vi "Delacor_lib_QMH_Check Loop Error.vi"(6 "Error Message Name (\"Error\")":string="Error", 9 "Ignore Errors":i32[](array[numeric]), 10 "error to process":errorcluster, 11 "Message Queue in":refnum<class "Delacor_lib_QMH_Message Queue.lvclass">) -> (2 "Enqueued Error?":bool, 3 "Message Queue out":refnum<class "Delacor_lib_QMH_Message Queue.lvclass">)   [LabVIEW 2024, in "Delacor_lib_QMH_Message Queue.lvclass"]
doc: "Check the 'error to process' to see if its code value matches any of the values in the 'Ignore Errors' array. If so, do nothing. If not, send an \"Error\" message containing the error data to the Message Handling Loop for further processing.\n____\nDQMH Framework: Palette 7.1.0.1503\nCopyright (c) 2025, DQMH Consortium"
uses:
  Delacor_lib_QMH_Message Queue.lvclass
  Delacor_lib_QMH_Message Queue.lvclass/Delacor_lib_QMH_Message Queue.ctl
  <vilib>/Delacor/Delacor QMH/Libraries/Message Queue_class/Delacor_lib_QMH_Enqueue Message (Single).vi
  Delacor_lib_QMH_Get Error Debug.vi
  Delacor_lib_QMH_Set Error Debug.vi
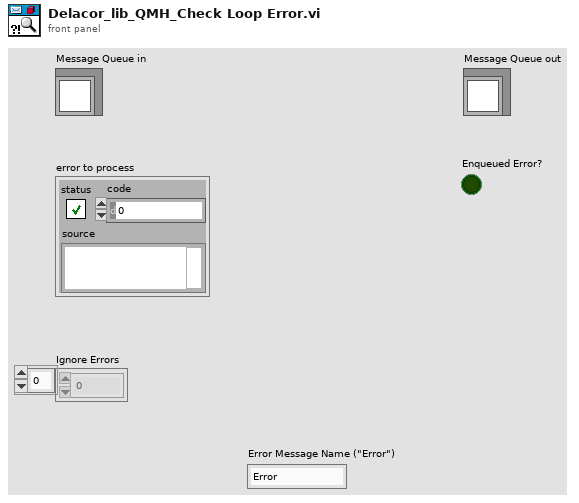
[diagram p1: front panel]
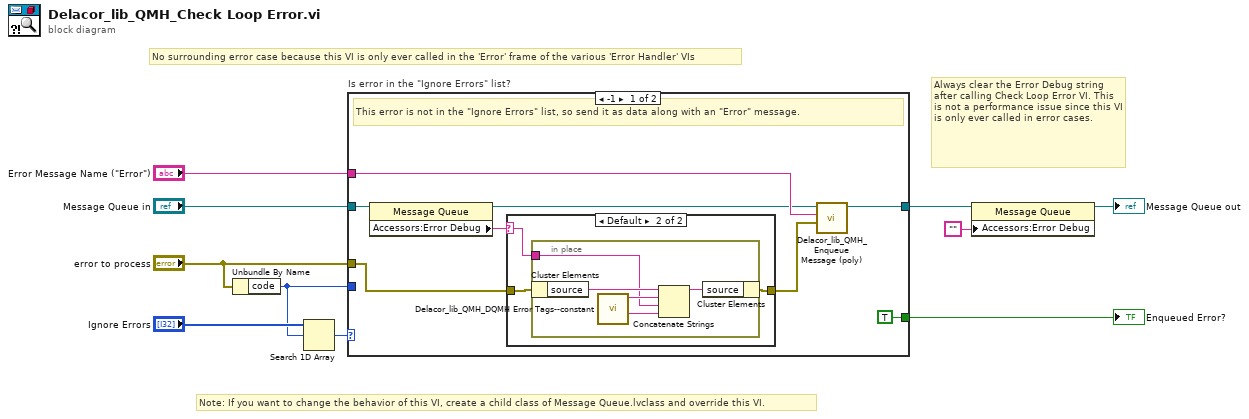
[diagram p0: block diagram]
diagram:
  # "No surrounding error case because this VI is only ever called in the 'Error' frame of the various 'Error Handler' VIs"
  # "Always clear the Error Debug string after calling Check Loop Error VI. This is not a performance issue since this VI is only ever called in error cases."
  # "Note: If you want to change the behavior of this VI, create a child class of Message Queue.lvclass and override this VI."
  n1 = Unbundle By Name("error to process") -> ("code"=w1:i32)
  n2 = Search 1D Array(1D array="Ignore Errors", element=w1) -> (index of element=w2:i32)  [unwired: 1 in]
  n3 = case "Is error in the \"Ignore Errors\" list?" shown="-1" w2 {
    tunnel: "error to process" -> [w14 _]
    tunnel: "Message Queue in" -> [w18 w28]
    tunnel: w1 -> [_ _]
    tunnel: [TRUE _] -> w7
    tunnel: [w16 w28] -> w6
    tunnel: "Error Message Name (\"Error\")" -> [w15 _]
    frame -1 {
      # "This error is not in the \"Ignore Errors\" list, so send it as data along with an \"Error\" message."
      n4 = property class="Message Queue"(reference=w18) -> (reference out=w11:refnum<class "Delacor_lib_QMH_Message Queue.lvclass">, "Accessors:Error Debug"=w12:string)  [unwired: 1 in, 1 out]
      n5 = case shown="Default" w12 {
        selector: w12 -> [_ w20]
        tunnel: w14 -> [w19 w22]
        tunnel: [w19 w21] -> w13
        frame "" {
          # "Don't add Error Debug string to error source string if it is empty."
        }
        frame Default {
          n6 = in-place {
            in-place-border: w20 -> [w24]
            n7 = in-place-cluster #1(w22) -> ("source"=w27:string)
            n8 = call <vilib>:"Delacor_lib_QMH_DQMH Error Tags--constant.vi"() -> ("Close Tag"=w23:string, "Open Tag"=w25:string)  [unwired: 10 in]
            n9 = Concatenate Strings(w27, w25, w24, w23) -> (w26:string)
            n10 = in-place-cluster #1("source"=w26) -> (w21:errorcluster)
          }
        }
      }
      n11 = call-poly <vilib>:"Delacor_lib_QMH_Enqueue Message (poly).vi"("Message Data"=w13, "Message"=w15, "Message Queue in"=w11) -> ("Message Queue out"=w16:refnum<class "Delacor_lib_QMH_Message Queue.lvclass">)  [unwired: 7 in, 1 out]
    }
    frame Default {
      # "This error is is in the \"Ignore Errors\" list, so do not send it for processing."
    }
  }
  "Enqueued Error?" <- w7
  n12 = property class="Message Queue"(reference=w6, "Accessors:Error Debug"="") -> (reference out=→"Message Queue out":refnum<class "Delacor_lib_QMH_Message Queue.lvclass">)  [unwired: 1 in, 1 out]
